vi "master.vi"(8 "ErrorIn":errorcluster, 11 "QueuesIn":T1) -> (0 "ErrorOut":errorcluster, 3 "QueuesOut":T1)   [LabVIEW 2019]
uses:
  utilities/Queues.ctl
  GUIVIs/GUIOutput.ctl
  MobileAnalyzer/mainVIs/analyzeAccelerationDataVIs/AnalyzedVibrationsData.ctl
  MobileAnalyzer/mainVIs/analyzeAccelerationDataVIs/AccelerationDataFrames.ctl
  MobileAnalyzer/mainVIs/analyzeAccelerationDataVIs/calculateFaultIndicatorsVIs/FaultDetections.ctl
  MobileAnalyzer/mainVIs/analyzeAccelerationDataVIs/calculateFaultIndicatorsVIs/ParameterFaultDetection.ctl
  MobileAnalyzer/mainVIs/analyzeAccelerationDataVIs/calculateFaultIndicatorsVIs/FaultParameter.ctl
  MobileAnalyzer/mainVIs/analyzeAccelerationDataVIs/calculateFaultIndicatorsVIs/FrequencyFaultDetection.ctl
  MobileAnalyzer/mainVIs/analyzeAccelerationDataVIs/calculateFaultIndicatorsVIs/OrdersFaultDetection.ctl
  masterVIs/Command.ctl
  MobileAnalyzer/mainVIs/TDMSmanagerVIs/TDMSAnalyzerData.ctl
  MobileAnalyzer/mainVIs/TDMSmanagerVIs/TDMSAnalyzerDataType.ctl
  saveAccelerationTimeDataToTDMSVIs/DataToSave.ctl
  masterVIs/CommandQueuesAction.ctl
  masterVIs/Thread.ctl
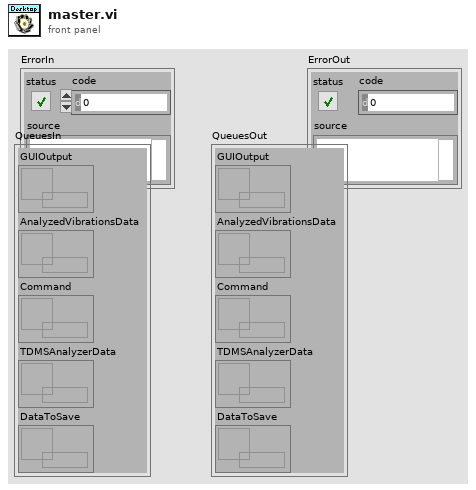
[diagram p1: front panel]
types:
  T1 = typedef "Queues.ctl" = cluster{"GUIOutput":refnum<queue>, "AnalyzedVibrationsData":refnum<queue>, "Command":refnum<queue>, "TDMSAnalyzerData":refnum<queue>, "DataToSave":refnum<queue>}
  T2 = typedef "CommandQueuesAction.ctl" = enum16{"Initialize", "Set", "Get", "ReleaseAll"}
  T3 = typedef "Command.ctl" = enum16{"None", "Connect", "Start", "Stop", "RestartAnalyzer", "Exit", "OpenDataFile", "CanBegin", "FileToSaveSettings", "AnalyzerSettings", "DownloadDataDialog", "DownloadData", "DeleteData"}
  T4 = typedef "Thread.ctl" = enum16{"GUI", "communicateWithAnalyzer", "saveDataToTDMS"}
  T5 = typedef "DesktopAppSettings.ctl" = cluster{"MobileAnalyzer IP":string, "Network Stream Timeout Code":i32, "Endpoint Destroyed Code":i32, "Save to file?":bool, "All threads":T4[], "Connected":bool, "AnalysisSettings":T6}
  T6 = typedef "AnalysisSettings.ctl" = cluster{"Fault Thresholds":T7, "Analysis series name":string, "Save data analysis?":bool, "Band size":i32, "OrderAnalysis?":bool, "Accelerometer":T9, "fs [Hz]":dbl}
  T7 = typedef "Thresholds.ctl" = cluster{"Parameters labels":T8[], "Parameters thresholds":dbl[], "Freqs and thresholds":dbl[][], "Orders and thresholds":dbl[][]}
  T8 = typedef "FaultParameter.ctl" = enum16{"Kurtosis", "RMS", "Crest factor"}
  T9 = typedef "Accelerometer.ctl" = enum16{"None", "MPU6050", "MMA7351"}
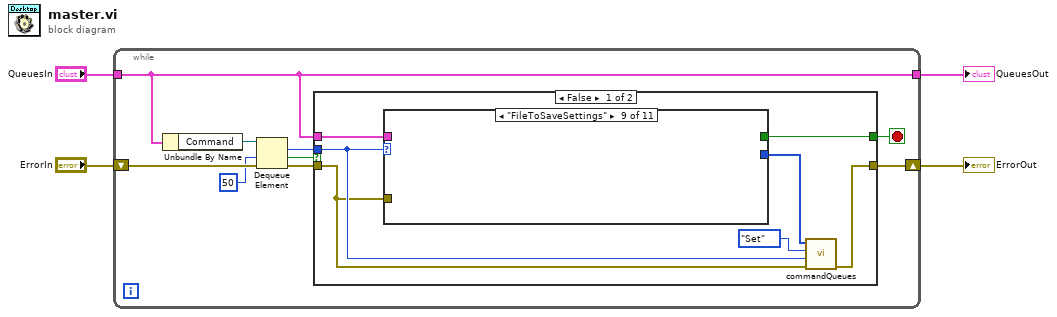
[diagram p0: block diagram]
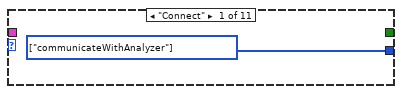
[diagram p2: hidden frame]
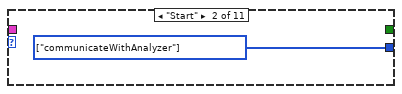
[diagram p3: hidden frame]
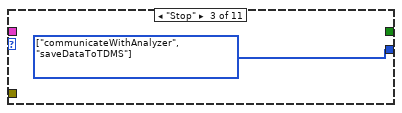
[diagram p4: hidden frame]
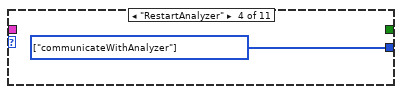
[diagram p5: hidden frame]
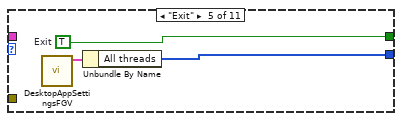
[diagram p6: hidden frame]
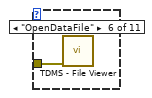
[diagram p7: hidden frame]
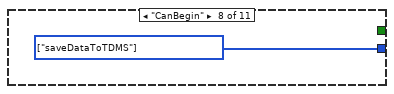
[diagram p9: hidden frame]
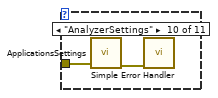
[diagram p10: hidden frame]
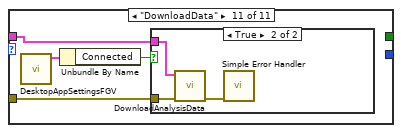
[diagram p11: hidden frame]
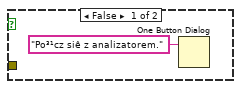
[diagram p12: hidden frame]
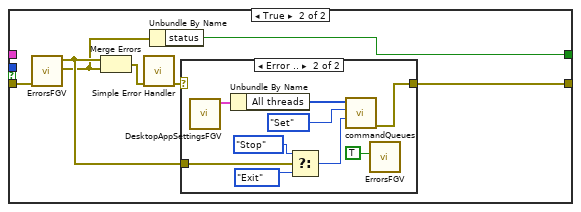
[diagram p13: hidden frame]
diagram:
  n1 = while {
    tunnel: "QueuesIn" -> [w5]
    shift-right: [w7] -> w2
    shift-left: "ErrorIn" -> [w12]
    tunnel: [w5] -> w1
    stop <- w6 stop-if-true
    n2 = Unbundle By Name(w5) -> ("Command"=w13:refnum<queue>)
    n3 = Dequeue Element(queue=w13, timeout in ms (-1)=50, error in (no error)=w12) -> (element=w8:T3, timed out?=w10:bool, error out=w9:errorcluster)  [unwired: 1 out]
    n4 = case shown="False" w10 {
      tunnel: w9 -> [w16 w44]
      tunnel: [w15 w46] -> w7
      tunnel: [w20 w41] -> w6
      tunnel: w8 -> [w17 _]
      tunnel: w5 -> [w14 _]
      frame False {
        n5 = case shown="\"FileToSaveSettings\"" w17 {
          tunnel: [_ _ _ _ w27 _ _ _ _ _ _] -> w20
          tunnel: [w21 w22 w23 w24 w25 _ _ w29 _ _ _] -> w19
          tunnel: w16 -> [_ _ _ _ _ w28 _ _ _ w31 w35]
          tunnel: w14 -> [_ _ _ _ _ _ _ _ _ _ w32]
          frame "Connect" {
            w21 = T4[] [enum."communicateWithAnalyzer"] items=["GUI", "communicateWithAnalyzer", "saveDataToTDMS"] ("Threads")
          }
          frame "Start" {
            w22 = T4[] [enum."communicateWithAnalyzer"] items=["GUI", "communicateWithAnalyzer", "saveDataToTDMS"] ("Threads")
          }
          frame "Stop" {
            w23 = T4[] [enum."communicateWithAnalyzer", enum."saveDataToTDMS"] items=["GUI", "communicateWithAnalyzer", "saveDataToTDMS"] ("Threads")
          }
          frame "RestartAnalyzer" {
            w24 = T4[] [enum."communicateWithAnalyzer"] items=["GUI", "communicateWithAnalyzer", "saveDataToTDMS"] ("Threads")
          }
          frame "Exit" {
            w27 = TRUE  # Exit
            n6 = call "DesktopAppSettingsFGV.vi"() -> ("DesktopAppSettingsOut"=w26:T5)  [unwired: 11 in]
            n7 = Unbundle By Name(w26) -> ("All threads"=w25:T4[])
          }
          frame "OpenDataFile" {
            n8 = call <vilib>:"TDMS - File Viewer.vi"("error in (no error)"=w28) -> ()  [unwired: 5 in, 2 out]
          }
          frame "None", Default {
          }
          frame "CanBegin" {
            w29 = T4[] [enum."saveDataToTDMS"] items=["GUI", "communicateWithAnalyzer", "saveDataToTDMS"] ("All threads")
          }
          frame "FileToSaveSettings" {
          }
          frame "AnalyzerSettings" {
            n9 = call "ApplicationsSettings.vi"("ErrorIn"=w31) -> ("ErrorOut"=w30:errorcluster)  [unwired: 10 in]
            n10 = call <vilib>:"Simple Error Handler.vi"("error in (no error)"=w30) -> ()  [unwired: 4 in, 5 out]
          }
          frame "DownloadData" {
            n11 = call "DesktopAppSettingsFGV.vi"() -> ("DesktopAppSettingsOut"=w34:T5)  [unwired: 11 in]
            n12 = Unbundle By Name(w34) -> ("Connected"=w33:bool)
            n13 = case shown="True" w33 {
              tunnel: w35 -> [_ w39]
              tunnel: w32 -> [_ w37]
              frame False {
                n14 = One Button Dialog(message="Po³¹cz siê z analizatorem.") -> ()  [unwired: 1 in, 1 out]
              }
              frame True {
                n15 = call "DownloadAnalysisData.vi"("ErrorIn"=w39, "QueuesIn"=w37) -> ("ErrorOut"=w38:errorcluster)  [unwired: 9 in]
                n16 = call <vilib>:"Simple Error Handler.vi"("error in (no error)"=w38) -> ()  [unwired: 4 in, 5 out]
              }
            }
          }
        }
        n17 = call "commandQueues.vi"("ErrorIn"=w16, "CommandIn"=w17, "CommandQueuesAction"=CommandQueuesAction."Set", "Threads"=w19) -> ("ErrorOut"=w15:errorcluster)  [unwired: 6 in, 1 out]
      }
      frame True {
        n18 = call "ErrorsFGV.vi"("CriticalErrorIn"=w44) -> ("GetCriticalError"=w42:errorcluster, "GetInternalError"=w43:errorcluster)  [unwired: 7 in, 2 out]
        n19 = Merge Errors(w43, w42) -> (w45:errorcluster)
        n20 = call <vilib>:"Simple Error Handler.vi"("error in (no error)"=w45) -> ("error out"=w40:errorcluster)  [unwired: 4 in, 4 out]
        n21 = Unbundle By Name(w42) -> ("status"=w41:bool)
        n22 = case shown="Error .." w40 {
          selector: w40 -> [w47 _]
          tunnel: [w47 w53] -> w46
          tunnel: w43 -> [_ w49]
          frame No Error {
          }
          frame Error {
            n23 = call "DesktopAppSettingsFGV.vi"() -> ("DesktopAppSettingsOut"=w55:T5)  [unwired: 11 in]
            n24 = Unbundle By Name(w55) -> ("All threads"=w54:T4[])
            n25 = Select(t=Command."Stop" ("CommandIn"), s=w49, f=Command."Exit") -> (s? t:f=w50:T3)
            n26 = call "commandQueues.vi"("CommandIn"=w50, "CommandQueuesAction"=CommandQueuesAction."Set", "Threads"=w54) -> ("ErrorOut"=w53:errorcluster)  [unwired: 7 in, 1 out]
            n27 = call "ErrorsFGV.vi"("Reset?"=TRUE) -> ()  [unwired: 7 in, 4 out]
          }
        }
      }
    }
  }
  "ErrorOut" <- w2
  "QueuesOut" <- w1
